vi "CThread State.vi"() -> (0 "Total VIs":i32=-1, 1 "Active?":bool)   [LabVIEW 2012, in "CThread.lvlib"]
uses:
  CThread.lvlib
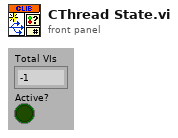
[diagram p1: front panel]
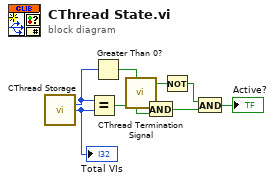
[diagram p0: block diagram]
diagram:
  n1 = call "CThread Storage.vi"() -> ("# VIs Initiated"=w7:i32, "Total VIs"=w6:i32)  [unwired: 10 in, 4 out]
  "Total VIs" <- w6
  n2 = Equal?(x=w7, y=w6) -> (x = y?=w4:bool)
  n3 = Greater Than 0?(x=w7) -> (x > 0?=w8:bool)
  n4 = call "CThread Termination Signal.vi"() -> ("Terminate?"=w2:bool)  [unwired: 5 in]
  n5 = And(x=w4, y=w8) -> (x .and. y?=w5:bool)
  n6 = Not(x=w2) -> (.not. x?=w1:bool)
  n7 = And(x=w1, y=w5) -> (x .and. y?=→"Active?":bool)
